vi "MAP Devices.vi"(8 "error in (no error)":errorcluster, 9 "CREAR":bool, 10 "BRAND SELECTED":enum16{"NXP", "CYPRESS", "SIMULATED"}(ring), 11 "Serial Devices in":refnum<class "Serial Devices.lvclass">) -> (0 "error out":errorcluster, 2 "VALOR":string, 3 "Serial Devices out":refnum<class "Serial Devices.lvclass">)   [LabVIEW 2019, in "Serial Devices.lvlib" / "Serial Devices.lvclass"]
uses:
  Serial Devices.lvclass
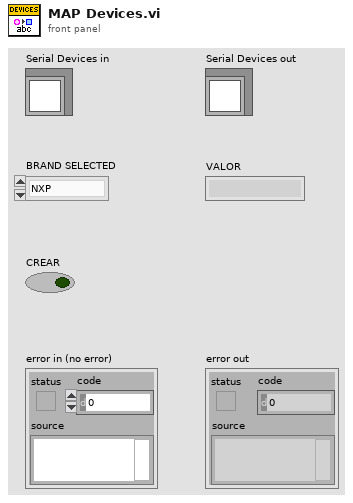
[diagram p1: front panel]
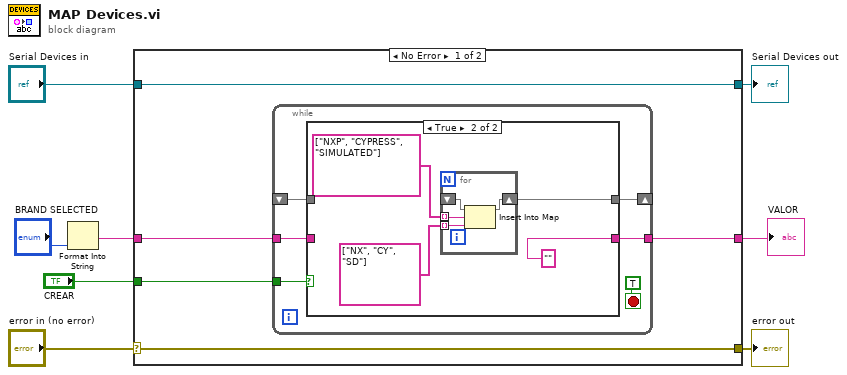
[diagram p0: block diagram]
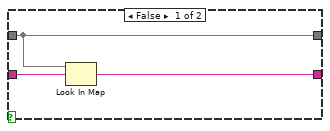
[diagram p2: hidden frame]
diagram:
  n1 = Format Into String("BRAND SELECTED") -> (resulting string=w1:string)  [unwired: 3 in, 1 out]
  n2 = case shown="No Error" "error in (no error)" {
    selector: "error in (no error)" -> [w12 w32]
    tunnel: [w12 w32] -> w7
    tunnel: [w13 w31] -> w5
    tunnel: "Serial Devices in" -> [w13 w31]
    tunnel: [w11 _] -> w4
    tunnel: "CREAR" -> [w10 _]
    tunnel: w1 -> [w9 _]
    frame No Error {
      n3 = while {
        shift-right: [w18] -> _
        shift-left: _ -> [w19]
        tunnel: w10 -> [w17]
        tunnel: [w16] -> w11
        tunnel: w9 -> [w14]
        stop <- TRUE stop-if-true
        n4 = case shown="True" w17 {
          tunnel: [w21 w26] -> w18
          tunnel: w19 -> [w21 _]
          tunnel: [w20 "" ("String")] -> w16
          tunnel: w14 -> [w22 _]
          frame False {
            n5 = Look In Map(map=w21, key=w22) -> (value=w20:string)  [unwired: 1 in, 1 out]
          }
          frame True {
            n6 = for {
              shift-right: [w30] -> w26
              shift-left: _ -> [w29]
              tunnel: string[] ["NXP", "CYPRESS", "SIMULATED"] -> [w28] mode=indexing
              tunnel: string[] ["NX", "CY", "SD"] -> [w27] mode=indexing
              n7 = Insert Into Map(map in=w29, key=w28, value=w27) -> (map out=w30:map{string, string})  [unwired: 2 out]
            }
          }
        }
      }
    }
    frame Error {
    }
  }
  "error out" <- w7
  "Serial Devices out" <- w5
  "VALOR" <- w4
